vi "create_full_token.vi"(0 "llm_openai_embedding in":refnum<class "llm_openai_embedding.lvclass">, 11 "error in (no error)":errorcluster) -> (4 "llm_openai_embedding out":refnum<class "llm_openai_embedding.lvclass">, 6 "header":string(combo)="Authorization", 8 "token":string, 15 "error out":errorcluster)   [LabVIEW 2020, in "llm_openai_embedding.lvclass"]
uses:
  llm_openai_embedding.lvclass
  llm_openai_embedding.lvclass/llm_openai_embedding.ctl
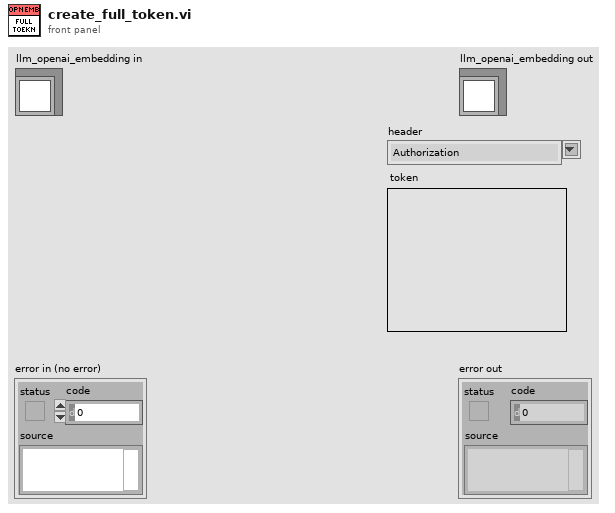
[diagram p1: front panel]
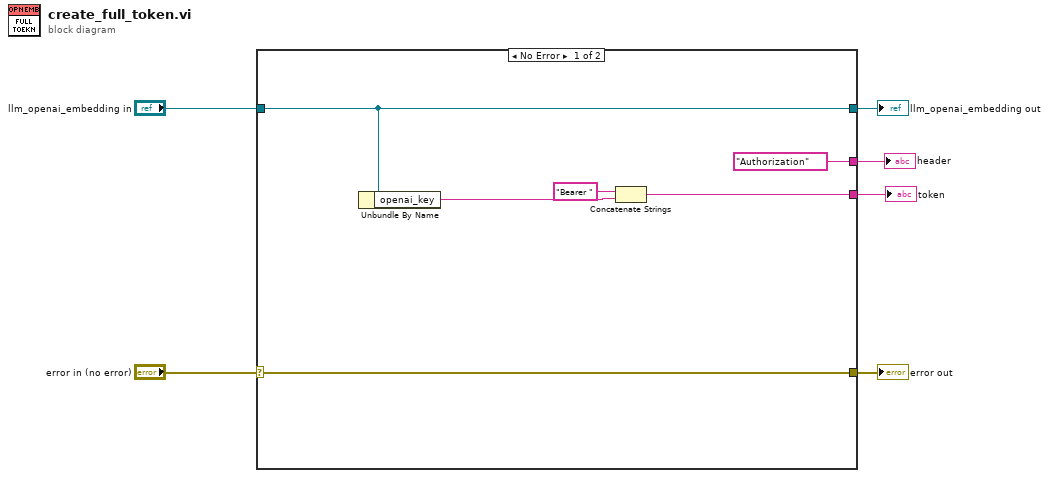
[diagram p0: block diagram]
diagram:
  n1 = case shown="No Error" "error in (no error)" {
    selector: "error in (no error)" -> [w12 w14]
    tunnel: [w12 w14] -> w5
    tunnel: [w9 w13] -> w3
    tunnel: "llm_openai_embedding in" -> [w9 w13]
    tunnel: ["Authorization" ("header") _] -> w2
    tunnel: [w7 _] -> w1
    frame No Error {
      n2 = Unbundle By Name(w9) -> ("openai_key"=w8:string)
      n3 = Concatenate Strings("Bearer " ("value"), w8) -> (w7:string)
    }
    frame Error {
    }
  }
  "error out" <- w5
  "llm_openai_embedding out" <- w3
  "token" <- w1
  "header" <- w2
